vi "Read data.vi"() -> ()   [LabVIEW 2021]
uses:
  <vilib>/Instr/_visa.llb/VISA Configure Serial Port (Instr).vi
panel:
  in  "stop\nstop":bool
  out "Magneticfield Z":dbl(graph)=-50.55
  out "Magneticfield Y":dbl(graph)=3.3
  out "Magneticfield X":dbl(graph)=-35.25
  out "Gyroscope Z":dbl(graph)=0.46
  out "Gyroscope Y":dbl(graph)=-0.23
  out "Gyroscope X":dbl(graph)=0.84
  out "Acceleration Z":dbl(graph)=-990.72
  out "Acceleration Y":dbl(graph)=-24.9
  out "Acceleration X":dbl(graph)=0.85
  out "array":dbl[](array[numeric])=[0.85, -24.9, -990.72, 0.84, -0.23, 0.46, -35.25, 3.3, -50.55]
  out "read buffer":string="0.85\t-24.90\t-990.72\t0.84\t-0.23\t0.46\t-35.25\t3.30\t-50.55\r\n"
  out "return count":u32=56
  out "error out":errorcluster
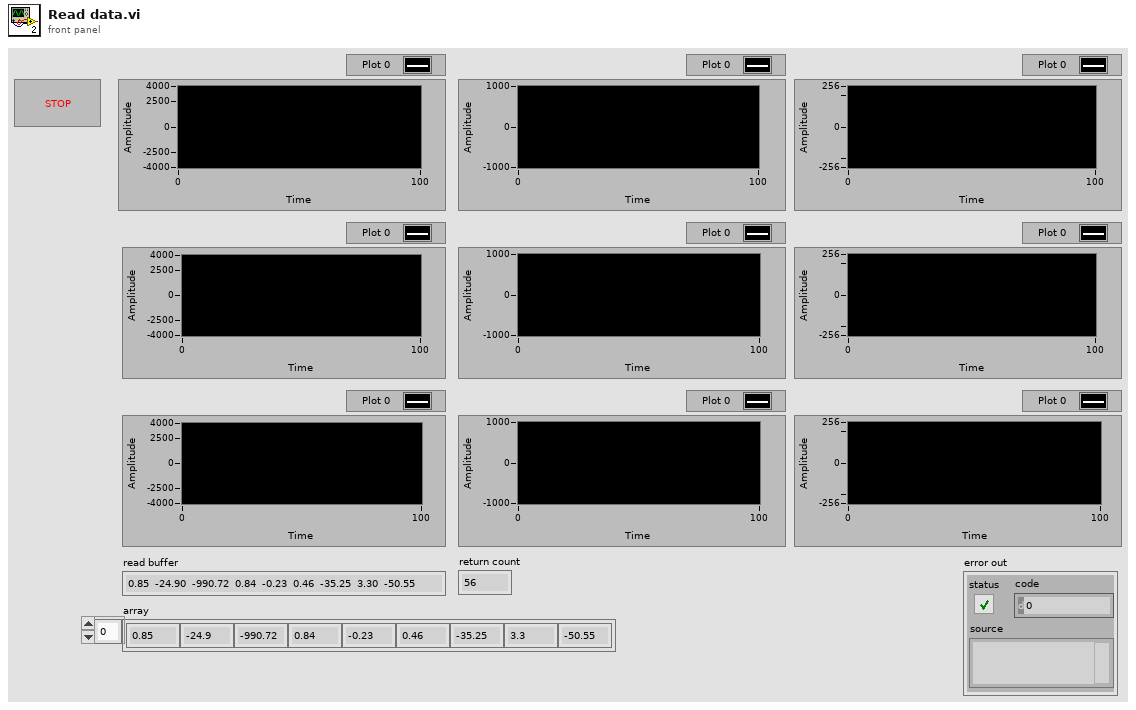
[diagram p1: front panel]
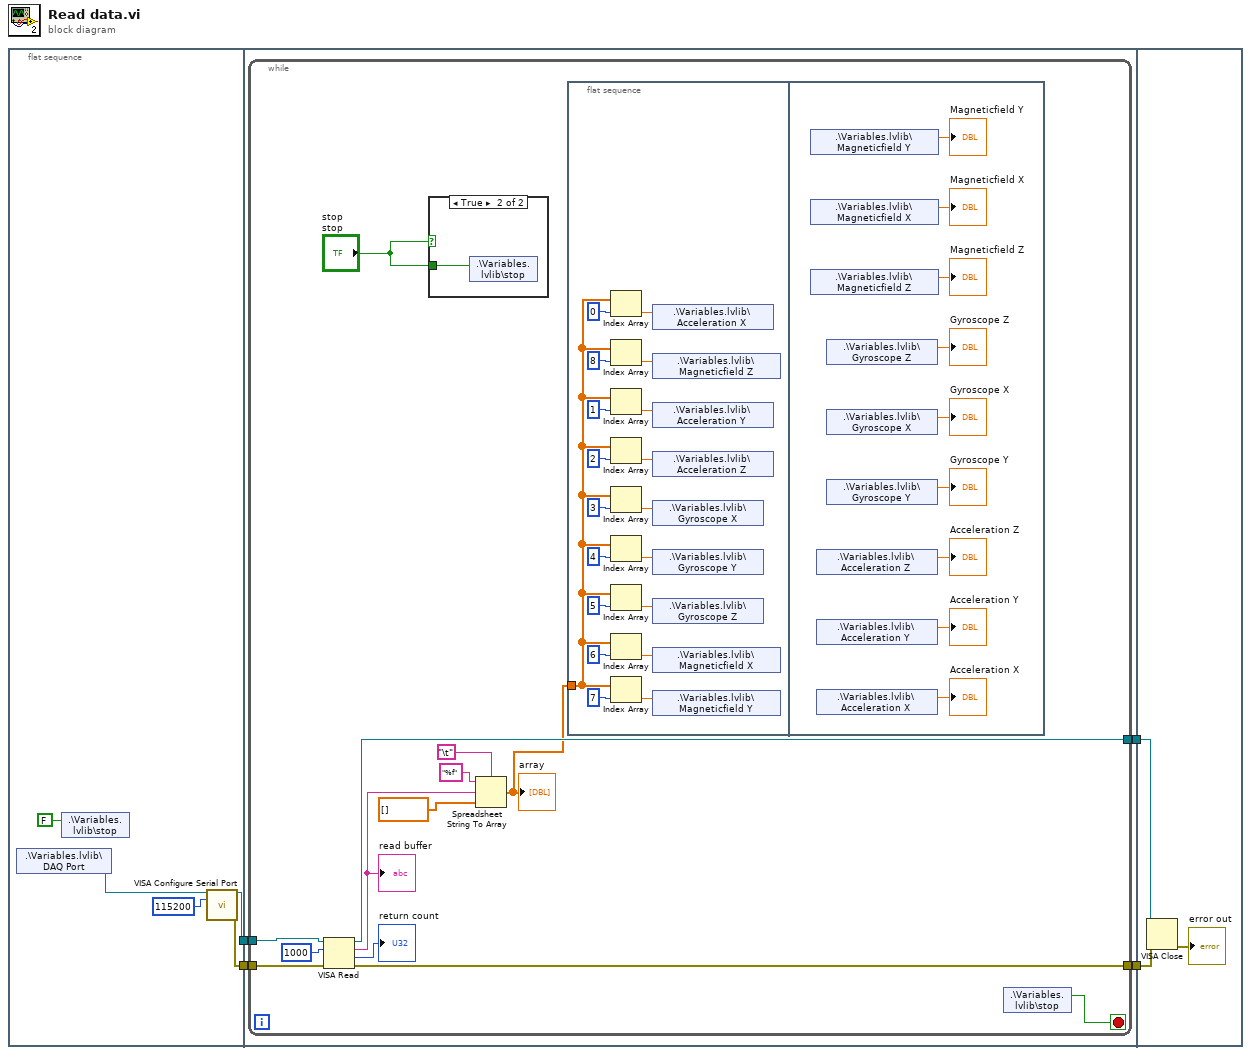
[diagram p0: block diagram]
diagram:
  n1 = flat-sequence {
    tunnel: [w6] -> w4
    tunnel: [w5] -> w3
    tunnel: w4 -> [w13]
    tunnel: w3 -> [w10]
    tunnel: [w12] -> w2
    tunnel: [w11] -> w1
    tunnel: w2 -> [w56]
    tunnel: w1 -> [w57]
    frame #0 {
      n2 = shared-variable ".\\Variables.lvlib\\DAQ Port"() -> (w9:refnum<visa-resource-name>)  [unwired: 1 in, 1 out]
      n3 = shared-variable ".\\Variables.lvlib\\stop"(FALSE ("stop")) -> ()  [unwired: 1 in, 1 out]
      n4 = call-poly "VISA Configure Serial Port"("VISA resource name"=w9, "baud rate (9600)"=u32 115200) -> ("VISA resource name out"=w6:refnum<visa-resource-name>, "error out"=w5:errorcluster)  [unwired: 12 in]
    }
    frame #1 {
      n5 = while {
        tunnel: w13 -> [w25]
        tunnel: [w24] -> w12
        tunnel: [w23] -> w11
        tunnel: w10 -> [w22]
        stop <- w16 stop-if-true
        n6 = VISA Read(VISA resource name=w25, byte count=u32 1000, error in (no error)=w22) -> (VISA resource name out=w24:refnum<visa-resource-name>, read buffer=w21:string, return count=→"return count":u32, error out=w23:errorcluster)
        "read buffer" <- w21
        n7 = case shown="True" "stop\nstop" {
          tunnel: "stop\nstop" -> [_ w27]
          frame False {
          }
          frame True {
            n8 = shared-variable ".\\Variables.lvlib\\stop"(w27) -> ()  [unwired: 1 in, 1 out]
          }
        }
        n9 = Spreadsheet String To Array(delimiter (Tab)="\t", format string="%f", spreadsheet string=w21, array type (2D Dbl)=dbl[] []) -> (array=w17:dbl[])
        "array" <- w17
        n10 = flat-sequence {
          tunnel: w17 -> [w37]
          frame #0 {
            n11 = Index Array(array=w37, index=0) -> (element=w36:dbl)
            n12 = Index Array(array=w37, index=8) -> (element=w35:dbl)
            n13 = Index Array(array=w37, index=1) -> (element=w34:dbl)
            n14 = Index Array(array=w37, index=2) -> (element=w33:dbl)
            n15 = Index Array(array=w37, index=3) -> (element=w32:dbl)
            n16 = Index Array(array=w37, index=4) -> (element=w31:dbl)
            n17 = Index Array(array=w37, index=5) -> (element=w30:dbl)
            n18 = Index Array(array=w37, index=6) -> (element=w29:dbl)
            n19 = Index Array(array=w37, index=7) -> (element=w28:dbl)
            n20 = shared-variable ".\\Variables.lvlib\\Acceleration X"(w36) -> ()  [unwired: 1 in, 1 out]
            n21 = shared-variable ".\\Variables.lvlib\\Magneticfield Z"(w35) -> ()  [unwired: 1 in, 1 out]
            n22 = shared-variable ".\\Variables.lvlib\\Acceleration Y"(w34) -> ()  [unwired: 1 in, 1 out]
            n23 = shared-variable ".\\Variables.lvlib\\Acceleration Z"(w33) -> ()  [unwired: 1 in, 1 out]
            n24 = shared-variable ".\\Variables.lvlib\\Gyroscope X"(w32) -> ()  [unwired: 1 in, 1 out]
            n25 = shared-variable ".\\Variables.lvlib\\Gyroscope Y"(w31) -> ()  [unwired: 1 in, 1 out]
            n26 = shared-variable ".\\Variables.lvlib\\Gyroscope Z"(w30) -> ()  [unwired: 1 in, 1 out]
            n27 = shared-variable ".\\Variables.lvlib\\Magneticfield X"(w29) -> ()  [unwired: 1 in, 1 out]
            n28 = shared-variable ".\\Variables.lvlib\\Magneticfield Y"(w28) -> ()  [unwired: 1 in, 1 out]
          }
          frame #1 {
            n29 = shared-variable ".\\Variables.lvlib\\Magneticfield Y"() -> (→"Magneticfield Y":dbl)  [unwired: 1 in, 1 out]
            n30 = shared-variable ".\\Variables.lvlib\\Magneticfield X"() -> (→"Magneticfield X":dbl)  [unwired: 1 in, 1 out]
            n31 = shared-variable ".\\Variables.lvlib\\Magneticfield Z"() -> (→"Magneticfield Z":dbl)  [unwired: 1 in, 1 out]
            n32 = shared-variable ".\\Variables.lvlib\\Acceleration Z"() -> (→"Acceleration Z":dbl)  [unwired: 1 in, 1 out]
            n33 = shared-variable ".\\Variables.lvlib\\Acceleration Y"() -> (→"Acceleration Y":dbl)  [unwired: 1 in, 1 out]
            n34 = shared-variable ".\\Variables.lvlib\\Acceleration X"() -> (→"Acceleration X":dbl)  [unwired: 1 in, 1 out]
            n35 = shared-variable ".\\Variables.lvlib\\Gyroscope Z"() -> (→"Gyroscope Z":dbl)  [unwired: 1 in, 1 out]
            n36 = shared-variable ".\\Variables.lvlib\\Gyroscope X"() -> (→"Gyroscope X":dbl)  [unwired: 1 in, 1 out]
            n37 = shared-variable ".\\Variables.lvlib\\Gyroscope Y"() -> (→"Gyroscope Y":dbl)  [unwired: 1 in, 1 out]
          }
        }
        n38 = shared-variable ".\\Variables.lvlib\\stop"() -> (w16:bool)  [unwired: 1 in, 1 out]
      }
    }
    frame #2 {
      n39 = VISA Close(VISA resource name=w56, error in (no error)=w57) -> (error out=→"error out":errorcluster)
    }
  }
